vi "KepcoDCPwr Max Number of Points.vi"(0 "VISA Session":refnum<visa-resource-name>, 5 "Model In":string, 7 "channel name (\"\")":string="\"\"", 11 "error in (no error)":errorcluster {"code" format="%.0x"}) -> (4 "VISA Session Out":refnum<visa-resource-name>, 6 "Model Out":string, 8 "channel name out (\"\")":string="\"\"" caption="channel name Out (\"\")", 10 "Max # of Pts":i32, 15 "error out":errorcluster {"code" format="%.0x"})   [LabVIEW 2013]
doc: "This VI resets the instrument and applies initial user specified settings from the Logical Name which was used to initialize the session. If the session was created without a Logical Name, this VI is equivalent to the KepcoDCPwr Reset.vi."
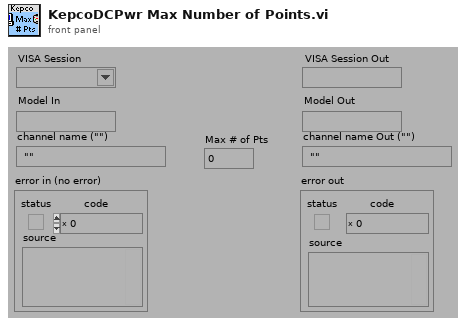
[diagram p1: front panel]
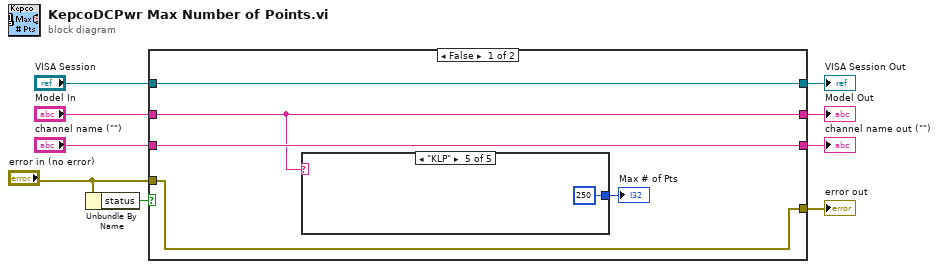
[diagram p0: block diagram]
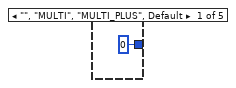
[diagram p2: hidden frame]
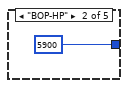
[diagram p3: hidden frame]
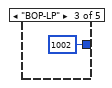
[diagram p4: hidden frame]
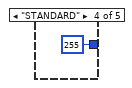
[diagram p5: hidden frame]
diagram:
  n1 = Unbundle By Name("error in (no error)") -> ("status"=w8:bool)
  n2 = case shown="False" w8 {
    tunnel: [w12 w23] -> w9
    tunnel: "error in (no error)" -> [w12 w23]
    tunnel: [w14 w22] -> w3
    tunnel: "VISA Session" -> [w14 w22]
    tunnel: [w11 w21] -> w2
    tunnel: "Model In" -> [w11 w21]
    tunnel: [w13 w20] -> w1
    tunnel: "channel name (\"\")" -> [w13 w20]
    frame False {
      n3 = case shown="\"KLP\"" w11 {
        tunnel: [0 5900 1002 255 250] -> w10
        frame "", "MULTI", "MULTI_PLUS", Default {
        }
        frame "BOP-HP" {
        }
        frame "BOP-LP" {
        }
        frame "STANDARD" {
        }
        frame "KLP" {
        }
      }
      "Max # of Pts" <- w10
    }
    frame True {
    }
  }
  "error out" <- w9
  "channel name out (\"\")" <- w1
  "VISA Session Out" <- w3
  "Model Out" <- w2
